vi "LedOpen (SubVI).vi"(8 "error in (no error)":errorcluster) -> (0 "error out":errorcluster, 3 "LedRef":refnum<class "Digital Output.lvclass">[](array[class]))   [LabVIEW 2020]
uses:
  <vilib>/CISH Robotics/L4VMX VMXpi/Digital Output/Digital Output.lvclass
  <vilib>/CISH Robotics/L4VMX VMXpi/Type Def/VMX Channel Index.ctl
  <vilib>/CISH Robotics/L4VMX VMXpi/L4VMX.lvlib
panel:
  # "19 Red Led\n20 Green Led"
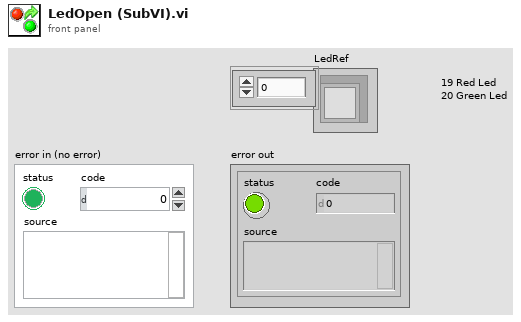
[diagram p1: front panel]
types:
  T1 = typedef "L4VMX.lvlib/VMX Channel Index.ctl" = enum16{"0", "1", "2", "3", "4", "5", "6", "7", "8", "9", "10", "11", "12", "13", "14", "15", "16", "17", "18", "19", "20", "21", "22", "23", "24", "25", "26", "27", "28", "29", "30", "31", "32", "33"}
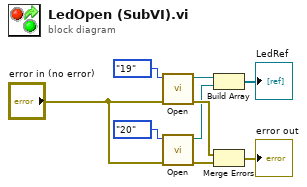
[diagram p0: block diagram]
diagram:
  n1 = call <vilib>:"Open.vi"("Error In"="error in (no error)", "VMX Channel Index"=VMX_Channel_Index."19") -> ("Error Out"=w7:errorcluster, "Digital Output Object"=w3:refnum<class "Digital Output.lvclass">)  [unwired: 8 in]
  n2 = call <vilib>:"Open.vi"("Error In"="error in (no error)", "VMX Channel Index"=VMX_Channel_Index."20") -> ("Error Out"=w8:errorcluster, "Digital Output Object"=w4:refnum<class "Digital Output.lvclass">)  [unwired: 8 in]
  n3 = Build Array(w3, w4) -> (→"LedRef":refnum<class "Digital Output.lvclass">[])
  n4 = Merge Errors(w7, w8) -> (→"error out":errorcluster)
